vi "Multiscale - Pyramids vs Wavelets Comparizon.vi"() -> ()   [LabVIEW 2023]
uses:
  Images/_Images.ctl
  <vilib>/vision/NI_Vision_Development_Module.lvlib
panel:
  out "Histogram Pyr":T1(graph)
  out "Pyramids Image":T2(plugin-control)
  out "Histogram Original":T1(graph)
  out "Histogram Wav":T1(graph)
  in  "Image":T3=enum."Part1"
  out "Wavelet Image":T2(plugin-control)
  out "Original Image":T2(plugin-control)
  # "Multoscale Contrast Enhancement Comparizon"
  # "Just run me. Advanced Signal Processing Toolkit is required!"
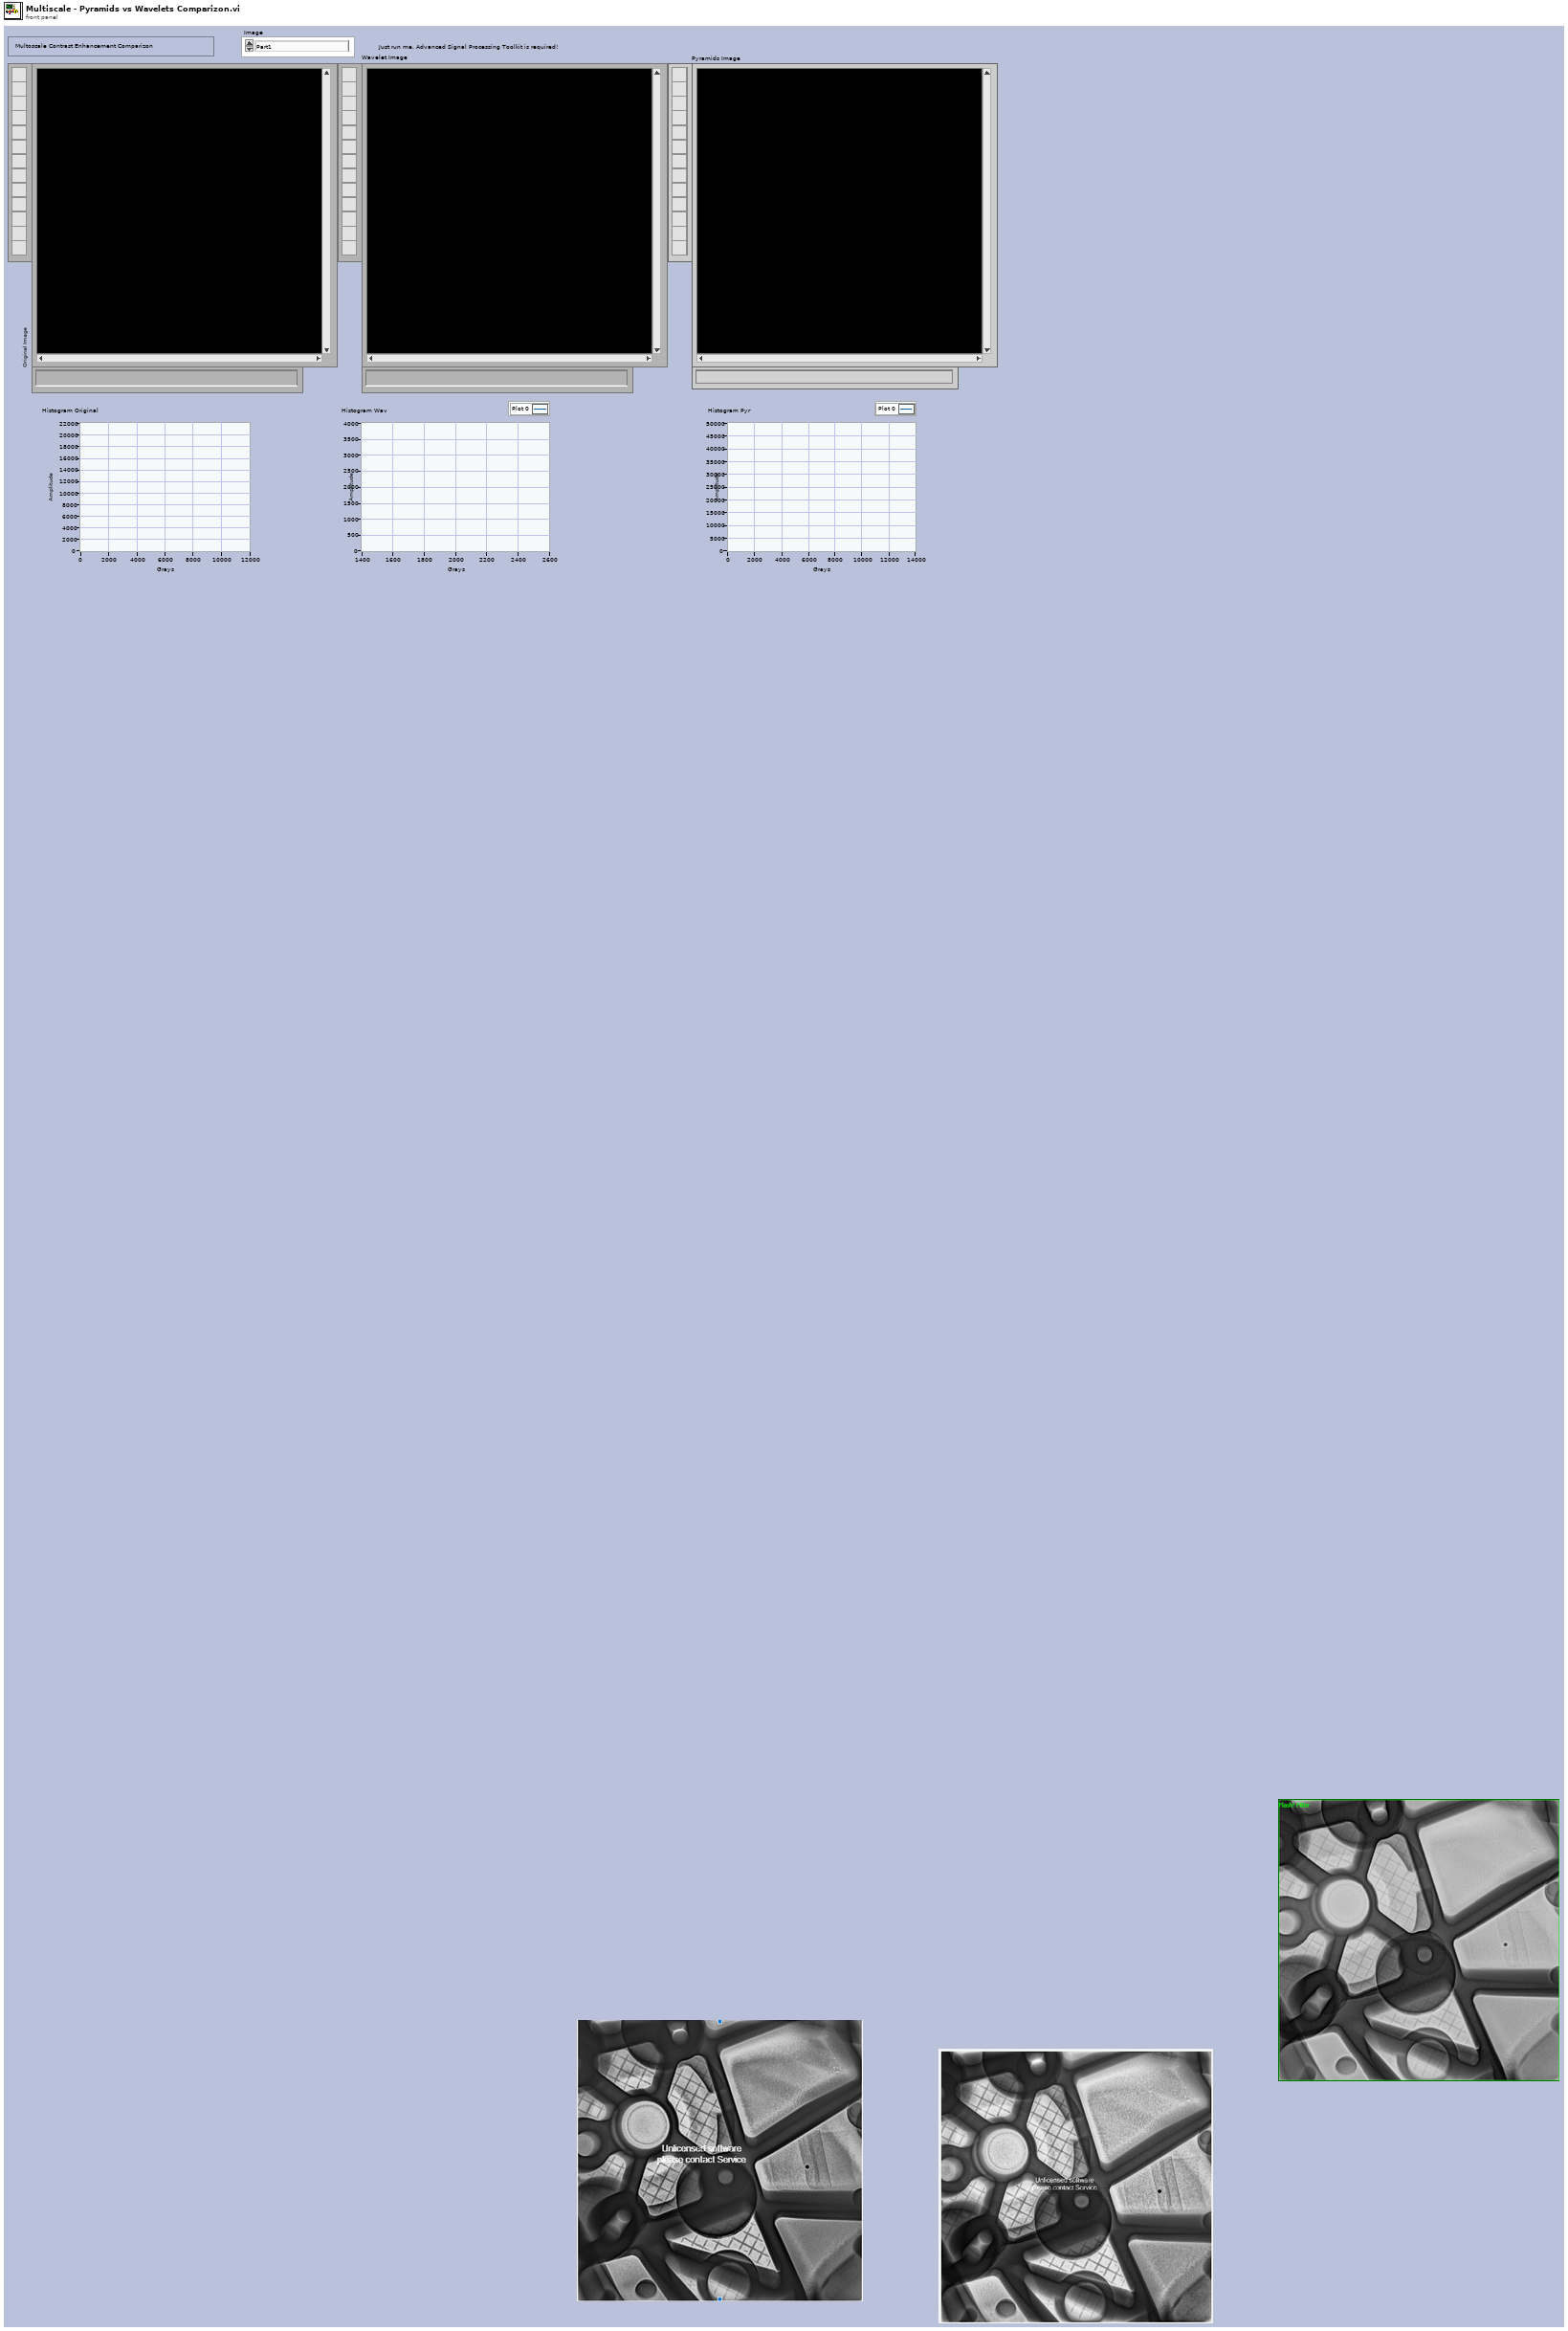
[diagram p1: front panel]
types:
  T1 = cluster{"Starting Value":sgl, "Incremental Value":sgl, "Histogram":u32[]}
  T2 = typedef "IMAQ Image.ctl" = refnum<image>
  T3 = typedef "_Images.ctl" = enum16{"Balls2", "Battery1", "Battery2", "Connector1", "Subwoofer1", "Subwoofer2", "Subwoofer3", "Subwoofer4", "Hase1", "Lamp1", "Lamp2", "Mouse1", "PhotoLens1", "Po1", "PowerSupply1", "Router", "--- Step Wedges ---", "Stepwedge1", "Stepwedge2", "Stepwedge3", "--- Fusion ---", "Fusion160kV", "Fusion2-120kV", "Fusion2-320kV", "Fusion300kV", "FusionPart1-120kV", "FusionPart1-180kV", "--- PART 01 ---", "Part1", "Part2", "Part3", "Part4", "Part5", "Part6", "Part7", "Part8", "--- Different Integrations ---", "Step2737-02Int", "Step2737-04Int", "Step2737-08Int", "Step2737-16Int", "Step2737-32Int", "Step2737-64Int"}
  T4 = typedef "Image Type" = u32
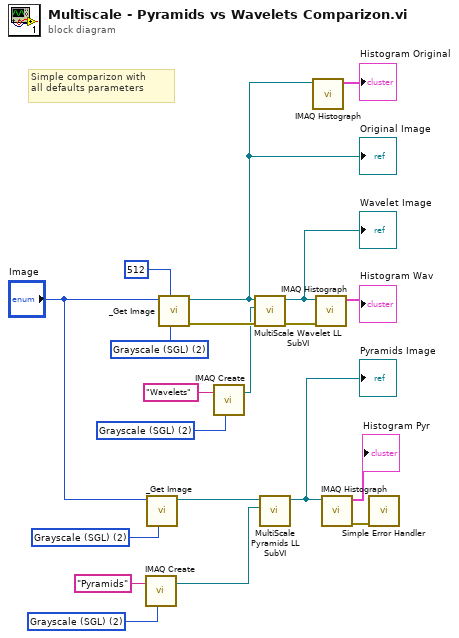
[diagram p0: block diagram]
diagram:
  w5 = T4 2 items=["Grayscale (U8)", "Grayscale (I16)", "Grayscale (SGL)", "Complex (CSG)", "RGB (U32)", "HSL (U32)", "RGB (U64)", "Grayscale (U16)"] ("Image Type (U16)")
  w9 = T4 2 items=["Grayscale (U8)", "Grayscale (I16)", "Grayscale (SGL)", "Complex (CSG)", "RGB (U32)", "HSL (U32)", "RGB (U64)", "Grayscale (U16)"] ("Image Type")
  w18 = T4 2 items=["Grayscale (U8)", "Grayscale (I16)", "Grayscale (SGL)", "Complex (CSG)", "RGB (U32)", "HSL (U32)", "RGB (U64)", "Grayscale (U16)"] ("Image Type (U16)")
  w19 = T4 2 items=["Grayscale (U8)", "Grayscale (I16)", "Grayscale (SGL)", "Complex (CSG)", "RGB (U32)", "HSL (U32)", "RGB (U64)", "Grayscale (U16)"] ("Image Type")
  # "Simple comparizon with\nall defaults parameters"
  n1 = call "IMAQ Create"("Image Name"="Pyramids", "Image Type"=w9) -> ("New Image"=w8:T2)  [unwired: 3 in, 1 out]
  n2 = call "_Get Image.vi"("Image Type (U16)"=w5, "Image"="Image") -> ("Image Out"=w4:T2)  [unwired: 6 in, 3 out]
  n3 = call "_Get Image.vi"("Image Type (U16)"=w18, "XY Resolution"=512, "Image"="Image") -> ("error out"=w15:errorcluster, "Image Out"=w3:T2)  [unwired: 5 in, 2 out]
  "Original Image" <- w3
  n4 = call "IMAQ Create"("Image Name"="Wavelets", "Image Type"=w19) -> ("New Image"=w14:T2)  [unwired: 3 in, 1 out]
  n5 = call "MultiScale Wavelet LL SubVI.vi"("error in (no error)"=w15, "Image Dst"=w14, "Image Src"=w3) -> ("error out"=w13:errorcluster, "Image Dst Out"=w2:T2)  [unwired: 7 in]
  "Wavelet Image" <- w2
  n6 = call "MultiScale Pyramids LL SubVI.vi"("Image Dst"=w8, "Image Src"=w4) -> ("Image Dst Out"=w1:T2)  [unwired: 8 in, 1 out]
  "Pyramids Image" <- w1
  n7 = call "IMAQ Histograph"("Image"=w3) -> ("Histogram Graph"=→"Histogram Original":T1)  [unwired: 7 in, 3 out]
  n8 = call "IMAQ Histograph"("error in (no error)"=w13, "Image"=w2) -> ("Histogram Graph"=→"Histogram Wav":T1)  [unwired: 6 in, 3 out]
  n9 = call "IMAQ Histograph"("Image"=w1) -> ("error out"=w11:errorcluster, "Histogram Graph"=→"Histogram Pyr":T1)  [unwired: 7 in, 2 out]
  n10 = call <vilib>:"Simple Error Handler.vi"("error in (no error)"=w11) -> ()  [unwired: 4 in, 5 out]
